vi "km_mile.vi"(0 "Viteza in Km":dbl(slide)=100.22026431718061 scale=0.0..250.0) -> (1 "Viteza in Km":dbl(knob)=100.22026431718061 scale=0.0..250.0, 2 "Viteza in mile":dbl(knob)=62.27398512507378 scale=0.0..200.0)   [LabVIEW 2009]
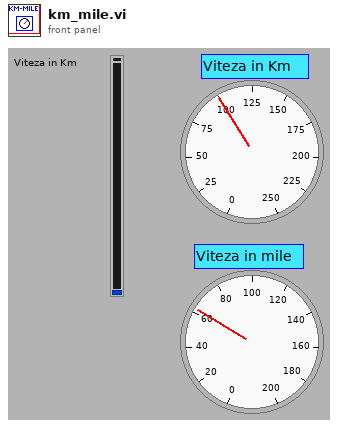
[diagram p1: front panel]
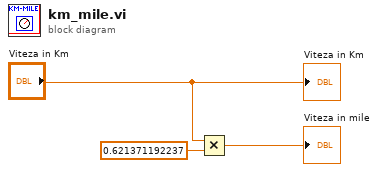
[diagram p0: block diagram]
diagram:
  n1 = Multiply(x="Viteza in Km", y=0.621371192237) -> (x*y=→"Viteza in mile":dbl)
  "Viteza in Km" <- "Viteza in Km"
